vi "Read INI file and trace graph.vi"(8 "error in (no error)":errorcluster, 9 "XY Graph in":cluster{"Value":dbl[], "Value":dbl[]}, 10 "This VI":refnum<vi>, 11 "Device Name":string) -> (0 "error out":errorcluster, 3 "XY Graph out":cluster{"Value":dbl[], "Value":dbl[]})   [LabVIEW 2013]
uses:
  <vilib>/Utility/file.llb/Read From Spreadsheet File (DBL).vi
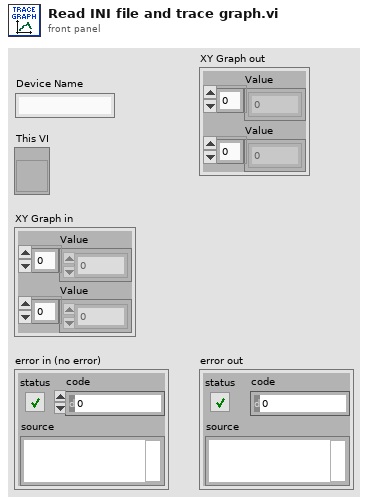
[diagram p1: front panel]
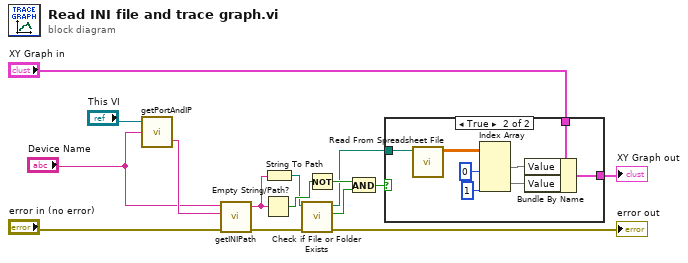
[diagram p0: block diagram]
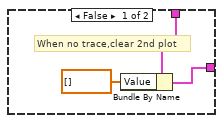
[diagram p2: hidden frame]
diagram:
  n1 = call "getPortAndIP.vi"("Device Name"="Device Name", "This Vi"="This VI") -> ("Device Type"=w10:string)  [unwired: 2 in, 4 out]
  n2 = call "getINIPath.vi"("error in (no error)"="error in (no error)", "DeviceType Name"=w10, "Device Name"="Device Name") -> ("error out"=→"error out":errorcluster, "reference trace path"=w3:string)  [unwired: 7 in]
  n3 = Empty String/Path?(string/path=w3) -> (empty?=w6:bool)
  n4 = String To Path(string=w3) -> (path=w4:path)
  n5 = call <vilib>:"Check if File or Folder Exists.vi"("path"=w4) -> ("file or folder exists?"=w8:bool, "dup path"=w5:path)  [unwired: 8 in, 1 out]
  n6 = Not(x=w6) -> (.not. x?=w7:bool)
  n7 = And(x=w7, y=w8) -> (x .and. y?=w9:bool)
  n8 = case shown="True" w9 {
    tunnel: "XY Graph in" -> [w17 w25]
    tunnel: [w16 w19] -> w14
    tunnel: w5 -> [_ w18]
    frame False {
      # "When no trace,clear 2nd plot"
      n9 = Bundle By Name(cluster=w17, "Value"=dbl[] []) -> (w16:cluster{"Value":dbl[], "Value":dbl[]})
    }
    frame True {
      n10 = call-poly <vilib>:"Read From Spreadsheet File.vi"("file path (dialog if empty)"=w18) -> ("all rows"=w24:dbl[][])  [unwired: 6 in, 4 out]
      n11 = Index Array(array=w24, index (col) #1=0 ("disabled index (col)"), index (col) #2=1 ("index (col)")) -> (element #1=w21:dbl[], element #2=w20:dbl[])  [unwired: 2 in]
      n12 = Bundle By Name(cluster=w25, "Value"=w21, "Value"=w20) -> (w19:cluster{"Value":dbl[], "Value":dbl[]})
    }
  }
  "XY Graph out" <- w14
